vi "BRig_dataExp_TPB_min_L.vi"() -> (2 "output_TPB_min_L":i32)   [LabVIEW 2014]
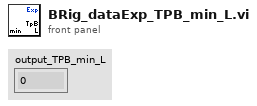
[diagram p1: front panel]
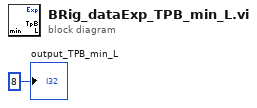
[diagram p0: block diagram]
diagram:
  "output_TPB_min_L" <- 8 ("output_iBlock")
